vi "Periodic Tasks.vi"(8 "error in":errorcluster) -> ()   [LabVIEW 2018]
doc: "This VI runs in parallel to other tasks. It can contain as many user-defined periodic loops as you need. These can carry out PID or other sorts of timed response."
uses:
  <vilib>/Rock Robotics/WPI/ThirdParty/Sensors/navX/_TypeDefs/FRIC_navX_DeviceNumbersTypeDef.ctl
  <vilib>/Rock Robotics/WPI/DriverStation/WPI_DriverStationRobotMode2.ctl
  <vilib>/Rock Robotics/WPI/Solenoid/WPI_SolenoidValue.ctl
  <vilib>/Rock Robotics/WPI/Utilities/WPI_GetSetVariantRefNum.vi
  Robot Global Data.vi
  <vilib>/addons/control/pid/pid.llb/PID Control Input Filter (DBL).vi
  <vilib>/Rock Robotics/Network Tables/NT Write Boolean.vi
  <vilib>/Rock Robotics/WPI/RobotDrive/WPI_RobotDriveArcadeDrive_Standard(NoSaturation).vi
  <vilib>/Rock Robotics/WPI/Solenoid/WPI_SolenoidSetEnum.vi
  <vilib>/regexp/Match Regular Expression.xnode
  <vilib>/addons/control/pid/NI_PID_pid.lvlib
  <vilib>/addons/control/pid/pid.llb/PID (DBL).vi
panel:
  out "element 5":bool
  out "element 4":bool
  out "element 3":bool
  out "element 2":bool
  in  "Stage2_Speed":dbl=0.75
  in  "Stage1_Speed":dbl=0.75
  in  "ElevatorLowerBounds":dbl
  in  "ElevatorUpperBoundes":dbl
  in  "RotationEncoder_TopBall":dbl format="%#_13g"
  in  "Stage2Encoder_TopBall":dbl format="%#_13g"
  in  "Stage1Encoder_TopBall":dbl format="%#_13g"
  in  "RotationEncoder_TopHatch":dbl format="%#_13g"
  in  "Stage2Encoder_TopHatch":dbl format="%#_13g"
  in  "Stage1Encoder_TopHatch":dbl format="%#_13g"
  in  "RotationEncoder_MedBall":dbl format="%#_13g"
  in  "Stage2Encoder_MedBall":dbl format="%#_13g"
  in  "Stage1Encoder_MedBall":dbl format="%#_13g"
  in  "RotationEncoder_MedHatch":dbl format="%#_13g"
  in  "Stage2Encoder_MedHatch":dbl format="%#_13g"
  in  "Stage1Encoder_MedHatch":dbl format="%#_13g"
  in  "RotationEncoder_CargoBall":dbl format="%#_13g"
  in  "Stage2Encoder_CargoBall":dbl format="%#_13g"
  in  "Stage1Encoder_CargoBall":dbl format="%#_13g"
  in  "RotationEncoder_LowRocketBall":dbl format="%#_13g"
  in  "Stage2Encoder_LowRocketBall":dbl format="%#_13g"
  in  "Stage1Encoder_LowRocketBall":dbl format="%#_13g"
  in  "RotationEncoder_LowHatch":dbl format="%#_13g"
  in  "Stage2Encoder_LowHatch":dbl format="%#_13g"
  in  "Stage1Encoder_LowHatch":dbl format="%#_13g"
  in  "RotationEncoder_StartPosition":dbl format="%#_13g"
  in  "Stage2Encoder_StartPosition":dbl format="%#_13g"
  in  "Stage1Encoder_StartPosition":dbl format="%#_13g"
  out "stage 1 encoder":dbl
  in  "Stage1_EncoderReset":bool
  in  "driveMultiplier":dbl=1.0
  in  "rotationMultiplier":dbl=0.7
  out "stage 2 encoder":dbl
  in  "Stage2_EnconderReset":bool
  out "YRPHfH":T1
  in  "Update":bool
  in  "Device Number":T2
  in  "Pug Mode":bool
  out "error out":errorcluster
  in  "Reset Enconder Arm":bool
  out "Arm Encoder":dbl
  in  "Shooter Speed":dbl
  # "Motor Speed Controls:"
  # "Arm Rotation Control Variable:"
  # "LIFT AND ARM CONTROLS:"
  # "DRIVE SYSTEMS:"
  # "Lift and Arm Encoder Positions"
  # "This is the multiplier associated with the drive train's forward and backwards speed. You want this number to be possitive and between 0 and 1"
  # "This is the multiplier associated with the drive train's rotation. You want this number to be possitive and between 0 and 1"
  # "PID Control for drivetrain. It would essentially act as\na stay put for the robot. This would, in theory, fight\nback against another robot's defense with equal force\nhelping to stablize the robot."
  # "TESTING:"
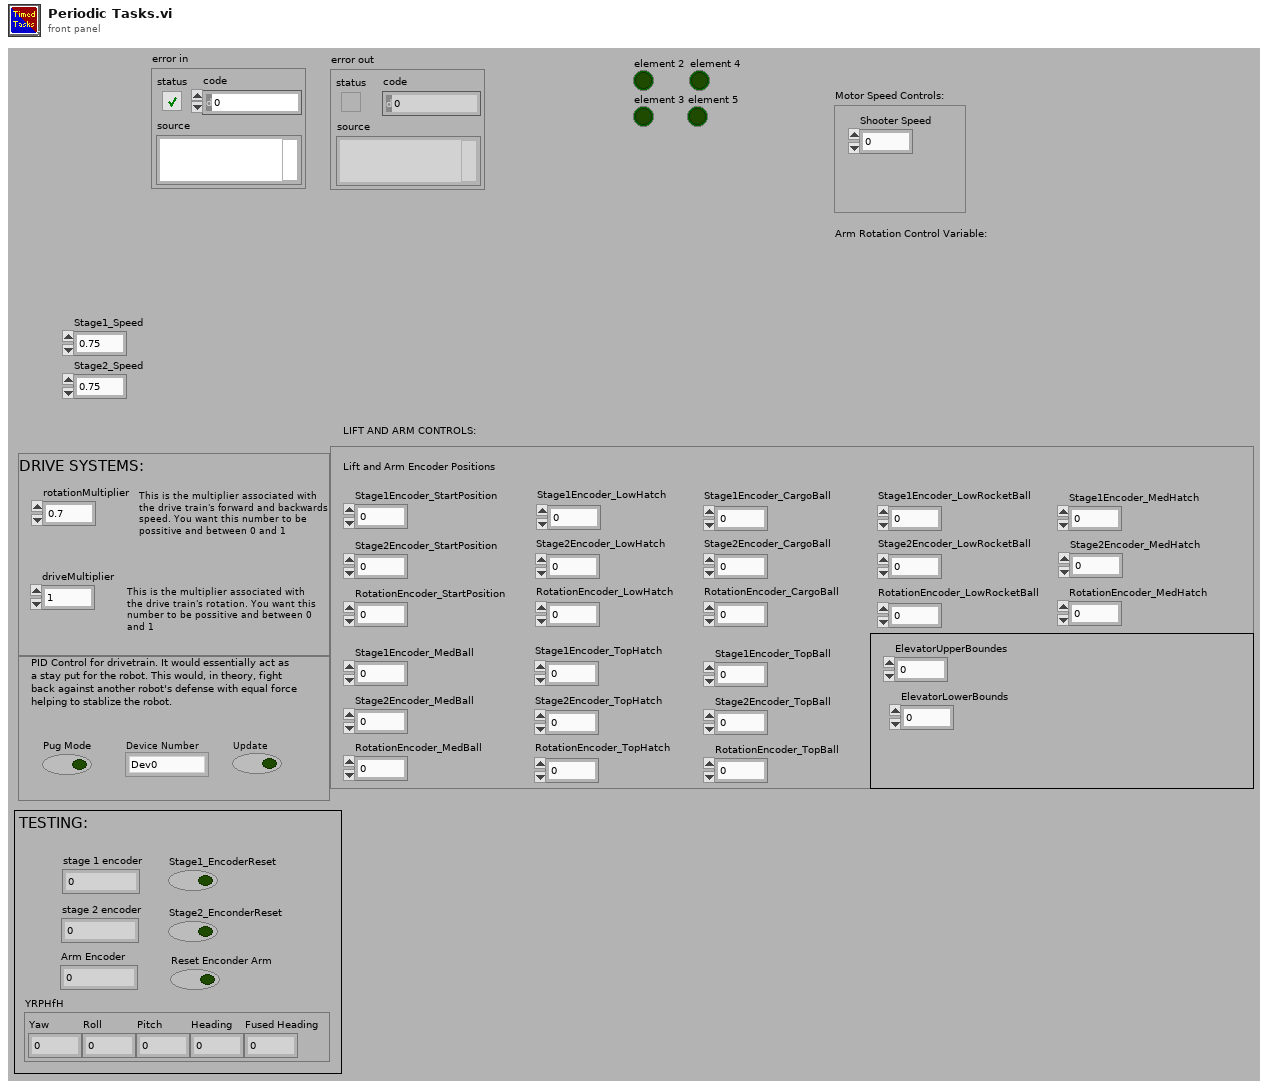
[diagram p1: front panel]
types:
  T1 = cluster{"Yaw":dbl, "Roll":dbl, "Pitch":dbl, "Heading":dbl, "Fused Heading":dbl}
  T2 = typedef "FRIC_navX_DeviceNumbersTypeDef.ctl" = enum16{"Dev0", "Dev1", "Dev2", "Dev3"}
  T3 = typedef "WPI_JoystickDevRef.ctl" = cluster{"Device":T4}
  T4 = typedef "WPI_JoystickDeviceEnum.ctl" = enum16{"USB 0", "USB 1", "USB 2", "USB 3", "USB 4", "USB 5"}
  T5 = typedef "WPI_RobotDriveDevRef.ctl" = cluster{"DevStatus":errorcluster, "Motors[]":T6[], "Square Inputs":bool, "Max Output":dbl}
  T6 = typedef "WPI_MotorControlDeviceRef.ctl" = cluster{"DeviceStatus":errorcluster, "Type":T7, "PWM":cluster{"PWM Channel":T8, "DeadBand":T9}, "CAN":cluster{"Device Number":u8, "SetOutput VI Ref":variant, "GetOutput VI Ref":variant, "Enable VI Ref":variant, "Disable VI Ref":variant, "Data":variant}, "Invert":bool, "DIO PWM":cluster{"PWM \"Enable\" Channel":T8, "DIOChannel":T10, "PWM Rate":dbl}}
  T7 = typedef "WPI_MotorControlType.ctl" = enum16{"PWM", "CAN", "DIO PWM"}
  T8 = typedef "FPGA_DIOPWMChannel.ctl" = enum8{"PWM 0", "PWM 1", "PWM 2", "PWM 3", "PWM 4", "PWM 5", "PWM 6", "PWM 7", "PWM 8", "PWM 9", "PWM MXP 0", "PWM MXP 1", "PWM MXP 2", "PWM MXP 3", "PWM MXP 4", "PWM MXP 5", "PWM MXP 6", "PWM MXP 7", "PWM MXP 8", "PWM MXP 9", "Invalid"}
  T9 = typedef "WPI_PWMDeadband.ctl" = cluster{"Name":string, "maxPositivePwm":i32, "minPositivePwm":i32, "centerPwm":i32, "maxNegativePwm":i32, "minNegativePwm":i32, "angularRange":u16}
  T10 = typedef "FPGA_DIOChannel.ctl" = enum8{"DIO 0", "DIO 1", "DIO 2", "DIO 3", "DIO 4", "DIO 5", "DIO 6", "DIO 7", "DIO 8", "DIO 9", "DIO MXP 0", "DIO MXP 1", "DIO MXP 2", "DIO MXP 3", "DIO MXP 4", "DIO MXP 5", "DIO MXP 6", "DIO MXP 7", "DIO MXP 8", "DIO MXP 9", "DIO MXP 10", "DIO MXP 11", "DIO MXP 12", "DIO MXP 13", "DIO MXP 14", "DIO MXP 15", "SPI Port CS1", "SPI Port CS2", "SPI Port CS3", "SPI Port MISO", "SPI Port MOSI", "Invalid"}
  T11 = typedef "WPI_EncoderDevRef.ctl" = cluster{"DevStatus":errorcluster, "EncoderIndex":T12, "CounterIndex":T13, "DistancePerCount":dbl, "Decoding Type":T14}
  T12 = typedef "FPGA_EncoderIdx.ctl" = enum8{"Enc 0", "Enc 1", "Enc 2", "Enc 3", "Enc 4", "Enc 5", "Enc 6", "Enc 7", "Invalid"}
  T13 = typedef "FPGA_CounterCtrSystemIndex.ctl" = enum8{"Ctr 0", "Ctr 1", "Ctr 2", "Ctr 3", "Ctr 4", "Ctr 5", "Ctr 6", "Ctr 7", "Invalid"}
  T14 = typedef "WPI_EncoderType.ctl" = enum16{"1x", "2x", "4x"}
  T15 = typedef "WPI_SolenoidDevRef.ctl" = cluster{"DevStatus":errorcluster, "Pneumatics Control Module":u8, "Forward Solenoid Channel":T16, "Reverse Solenoid Channel":T16}
  T16 = typedef "WPI_SolenoidChannel.ctl" = enum8{"Solenoid 0", "Solenoid 1", "Solenoid 2", "Solenoid 3", "Solenoid 4", "Solenoid 5", "Solenoid 6", "Solenoid 7", "Invalid"}
  T17 = typedef "WPI_DriverStationRobotMode2.ctl" = enum16{"Autonomous Disabled", "Autonomous Enabled", "Teleop Disabled", "Teleop Enabled", "Disconnected", "Finish", "Test Disabled", "Test Enabled", "Emergency Stopped"}
  T18 = typedef "WPI_SolenoidValue.ctl" = enum16{"Off", "On", "Forward", "Reverse"}
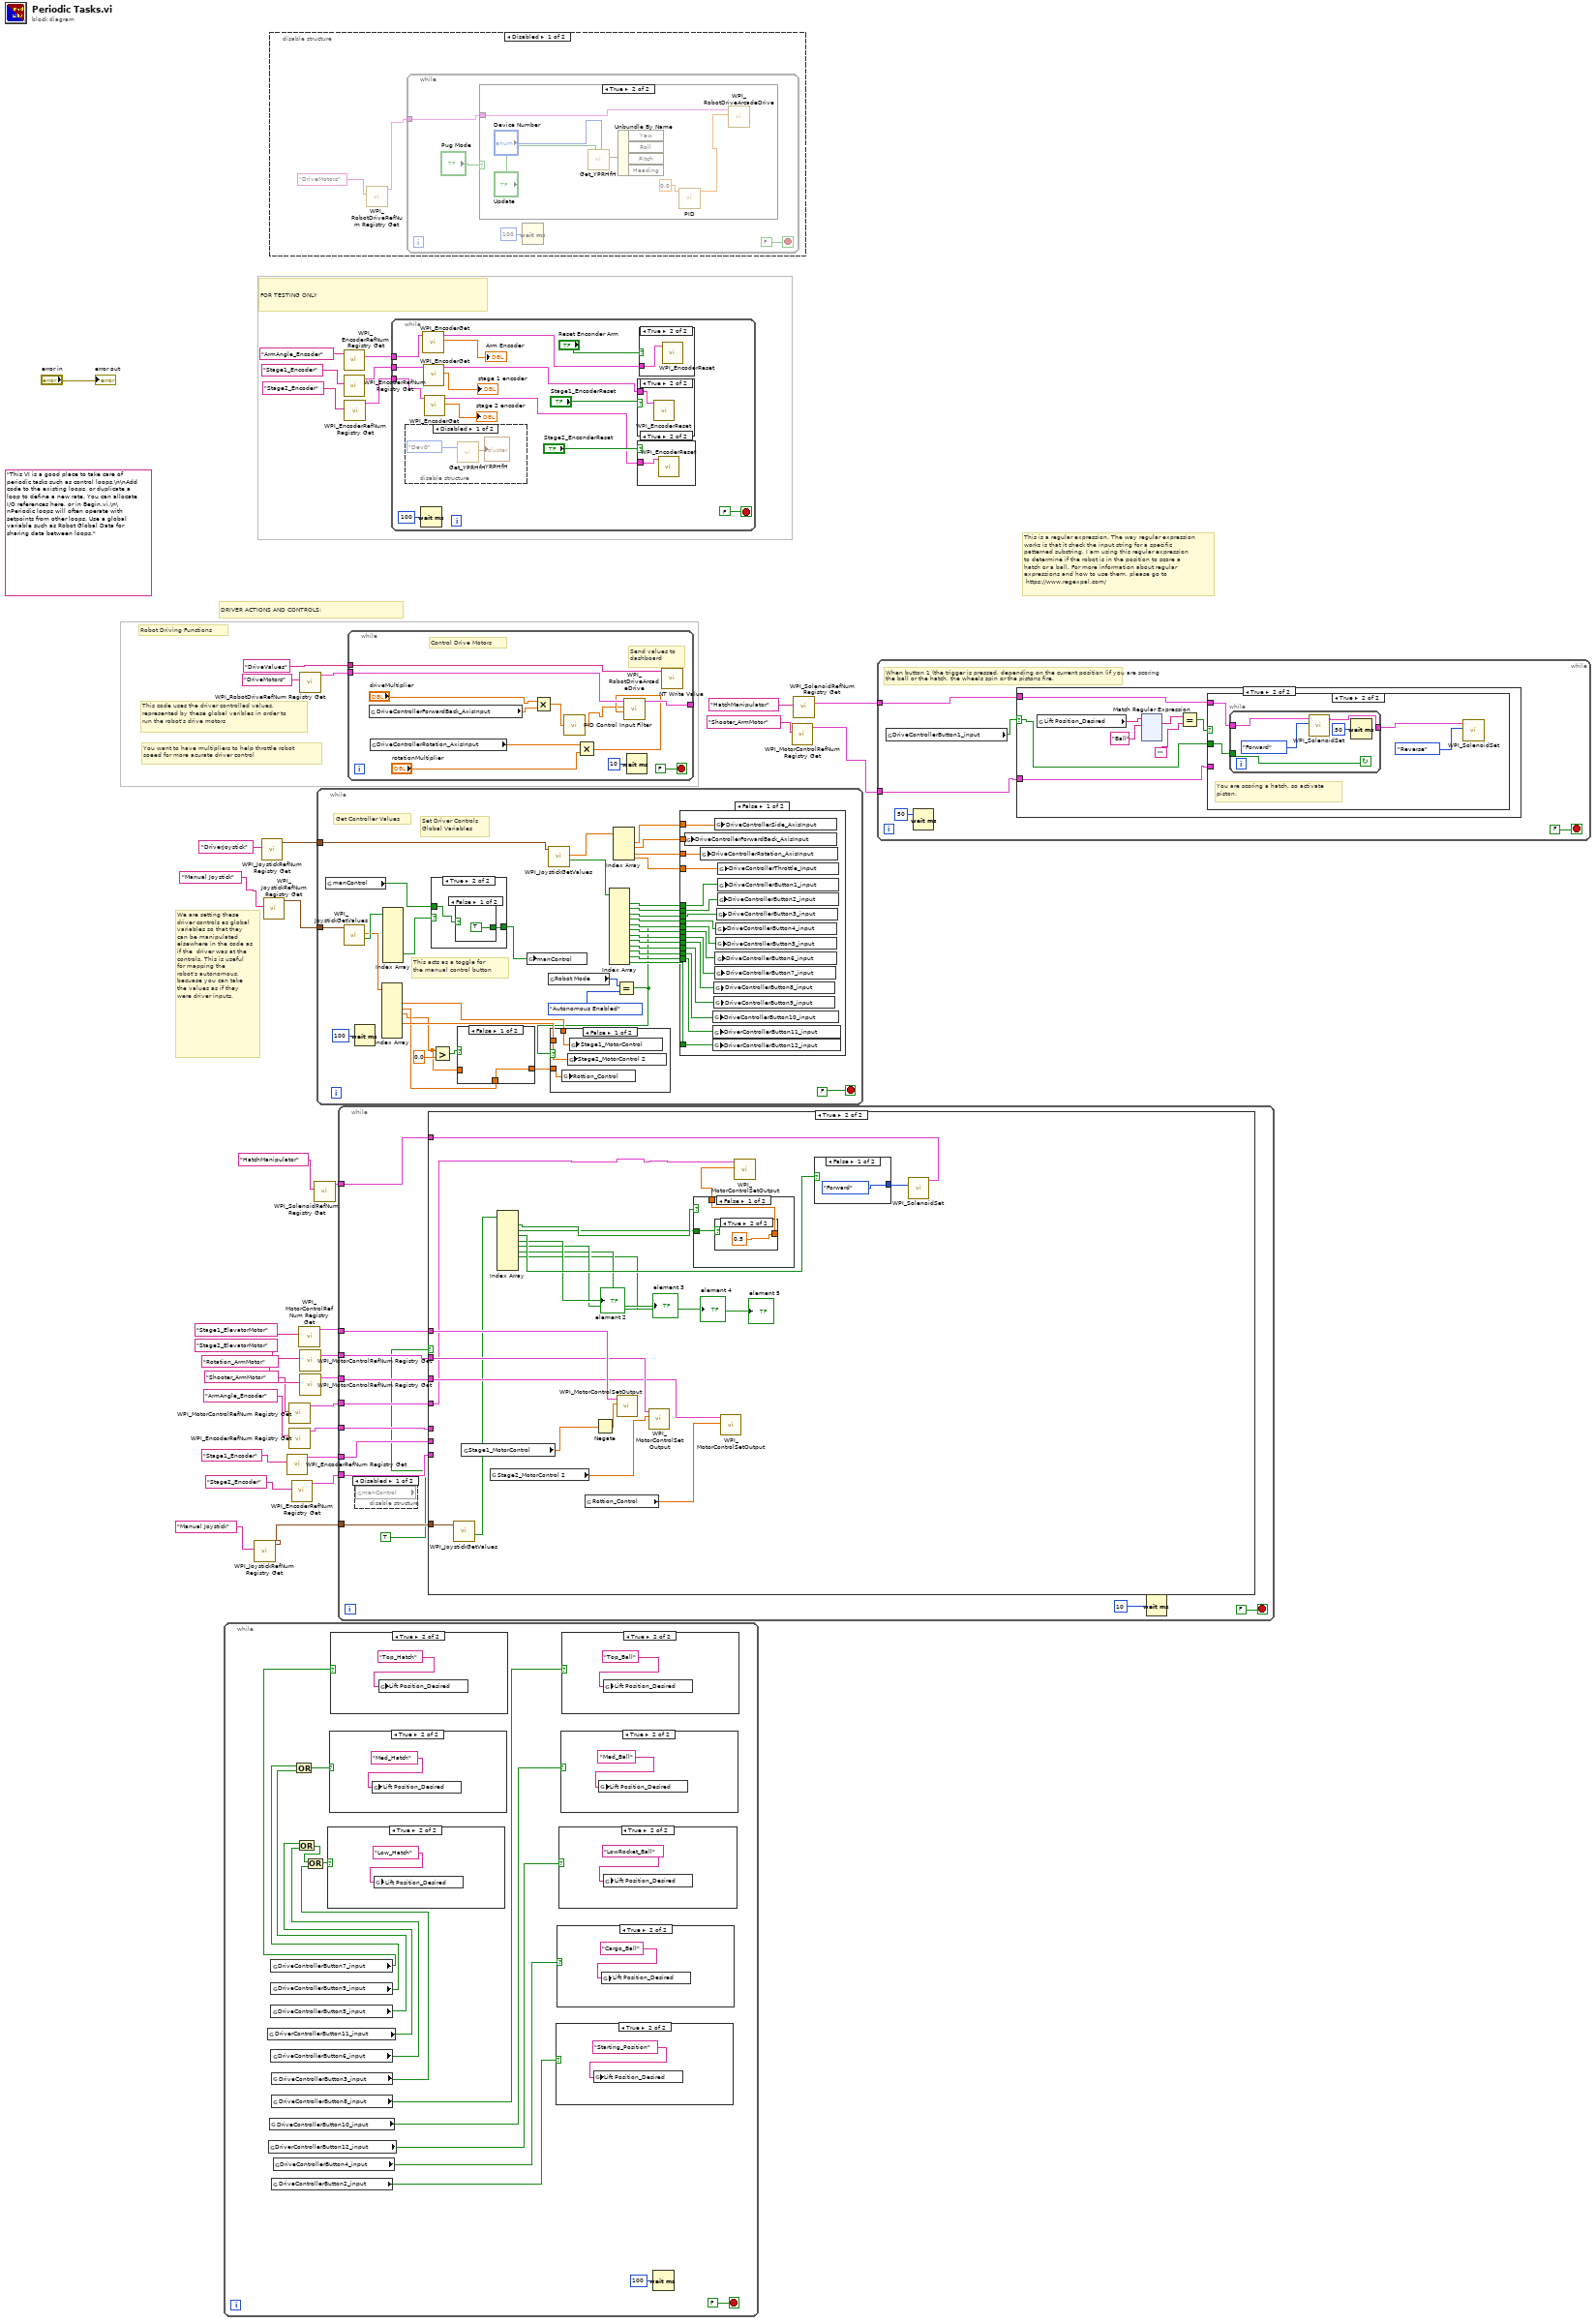
[diagram p0: block diagram]
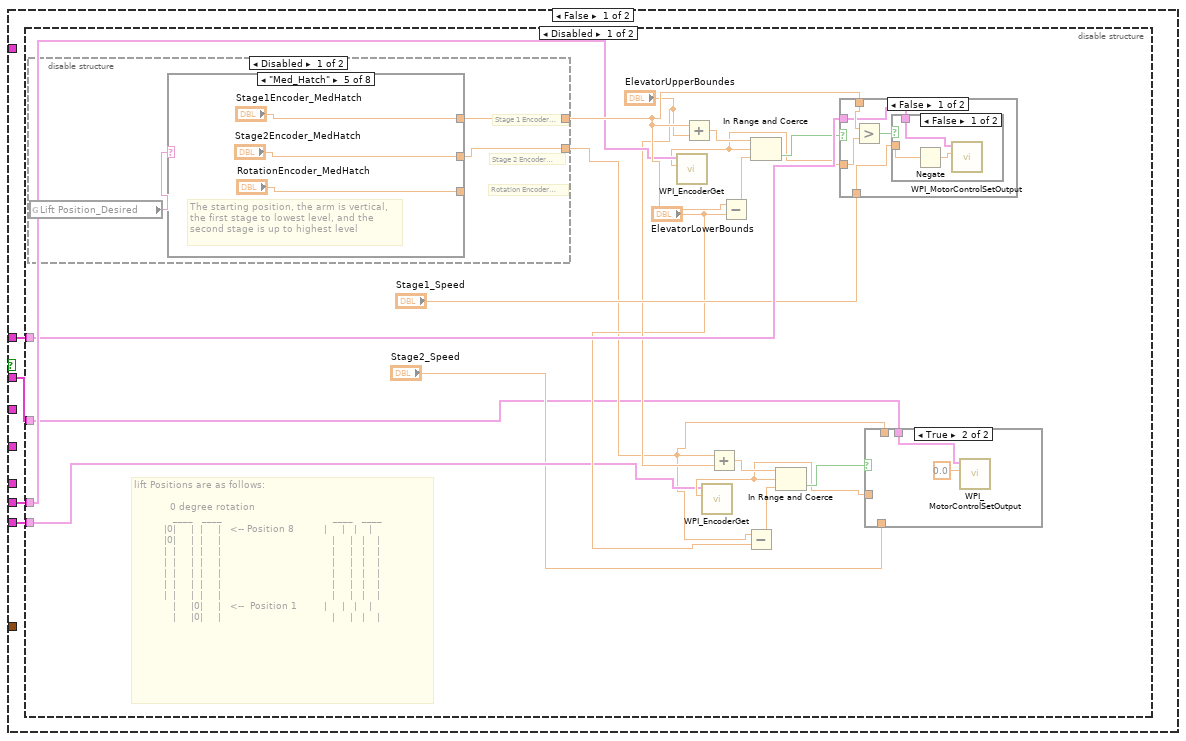
[diagram p3: hidden frame]
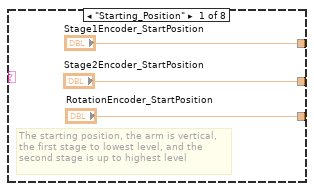
[diagram p4: hidden frame]
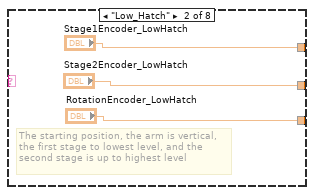
[diagram p5: hidden frame]
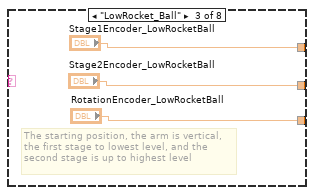
[diagram p6: hidden frame]
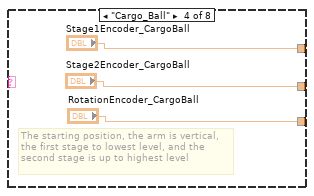
[diagram p7: hidden frame]
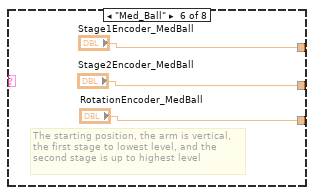
[diagram p8: hidden frame]
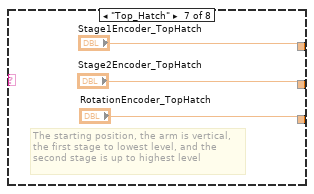
[diagram p9: hidden frame]
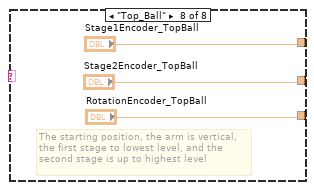
[diagram p10: hidden frame]
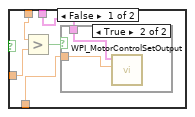
[diagram p12: hidden frame]
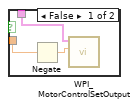
[diagram p13: hidden frame]
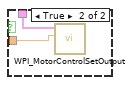
[diagram p14: hidden frame]
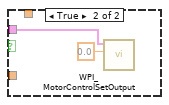
[diagram p15: hidden frame]
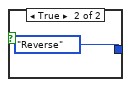
[diagram p17: hidden frame]
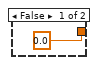
[diagram p18: hidden frame]
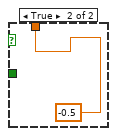
[diagram p19: hidden frame]
diagram:
  (unwired) "This VI is a good place to take care of periodic tasks such as control loops.\n\nAdd code to the existing loops, or duplicate a loop to define a new rate. You can allocate I/O references here, or in Begin.vi.\n\nPeriodic loops will often operate with setpoints from other loops. Use a global variable such as Robot Global Data for sharing data between loops."
  # "We are setting these driver controls as global variables so that they can be manipulated elsewhere in the code as if the  driver was at the controls. This is useful for mapping the\nrobot's autonomous, becuase you can take\nthe values as if they were driver inputs."
  # "You want to have multipliers to help throttle robot\nsoeed for more acurate driver control"
  # "This code uses the driver controlled values,\nrepresented by these global varibles in order to\nrun the robot's drive motors"
  # "FOR TESTING ONLY"
  # "This is a regular expression. The way regular expression\nworks is that it check the input string for a specific\npatterned substring. I am using this regular expression\nto determine if the robot is in the position to score a \nhatch or a ball. For more information about regular\nexpressions and how to use them, please go to\n https://www.regexpal.com/"
  # "Robot Driving Functions"
  # "DRIVER ACTIONS AND CONTROLS:"
  n1 = while {
    stop <- FALSE stop-if-true
    n2 = global read "Robot Global Data.vi" "DriverControllerButton11_input"() -> (w47:bool)
    n3 = global read "Robot Global Data.vi" "DriverControllerButton12_input"() -> (w41:bool)
    n4 = global read "Robot Global Data.vi" "DriveControllerButton10_input"() -> (w42:bool)
    n5 = global read "Robot Global Data.vi" "DriveControllerButton7_input"() -> (w51:bool)
    n6 = global read "Robot Global Data.vi" "DriveControllerButton9_input"() -> (w49:bool)
    n7 = global read "Robot Global Data.vi" "DriveControllerButton5_input"() -> (w48:bool)
    n8 = global read "Robot Global Data.vi" "DriveControllerButton6_input"() -> (w46:bool)
    n9 = global read "Robot Global Data.vi" "DriveControllerButton3_input"() -> (w37:bool)
    n10 = global read "Robot Global Data.vi" "DriveControllerButton8_input"() -> (w43:bool)
    n11 = global read "Robot Global Data.vi" "DriveControllerButton2_input"() -> (w44:bool)
    n12 = global read "Robot Global Data.vi" "DriveControllerButton4_input"() -> (w40:bool)
    n13 = Or(x=w49, y=w48) -> (x .or. y?=w50:bool)
    n14 = Or(x=w47, y=w46) -> (x .or. y?=w38:bool)
    n15 = Or(x=w38, y=w37) -> (x .or. y?=w45:bool)
    n16 = case shown="True" w45 {
      frame False {
      }
      frame True {
        n17 = global write "Robot Global Data.vi" "Lift Position_Desired"("Low_Hatch") -> ()
      }
    }
    n18 = case shown="True" w50 {
      frame False {
      }
      frame True {
        n19 = global write "Robot Global Data.vi" "Lift Position_Desired"("Med_Hatch") -> ()
      }
    }
    n20 = case shown="True" w51 {
      frame False {
      }
      frame True {
        n21 = global write "Robot Global Data.vi" "Lift Position_Desired"("Top_Hatch") -> ()
      }
    }
    n22 = case shown="True" w44 {
      frame False {
      }
      frame True {
        n23 = global write "Robot Global Data.vi" "Lift Position_Desired"("Starting_Position") -> ()
      }
    }
    n24 = case shown="True" w40 {
      frame False {
      }
      frame True {
        n25 = global write "Robot Global Data.vi" "Lift Position_Desired"("Cargo_Ball") -> ()
      }
    }
    n26 = case shown="True" w41 {
      frame False {
      }
      frame True {
        n27 = global write "Robot Global Data.vi" "Lift Position_Desired"("LowRocket_Ball") -> ()
      }
    }
    n28 = case shown="True" w42 {
      frame False {
      }
      frame True {
        n29 = global write "Robot Global Data.vi" "Lift Position_Desired"("Med_Ball") -> ()
      }
    }
    n30 = case shown="True" w43 {
      frame False {
      }
      frame True {
        n31 = global write "Robot Global Data.vi" "Lift Position_Desired"("Top_Ball") -> ()
      }
    }
    n32 = Wait (ms)(milliseconds to wait=u32 100) -> ()  [unwired: 1 out]
  }
  n33 = call <vilib>:"WPI_JoystickRefNum Registry Get.vi"("refnum name"="Manual Joystick") -> ("JoystickDevRef"=w24:T3)  [unwired: 9 in, 1 out]
  n34 = call <vilib>:"WPI_JoystickRefNum Registry Get.vi"("refnum name"="DriverJoystick") -> ("JoystickDevRef"=w32:T3)  [unwired: 9 in, 1 out]
  n35 = call <vilib>:"WPI_JoystickRefNum Registry Get.vi"("refnum name"="Manual Joystick") -> ("JoystickDevRef"=w21:T3)  [unwired: 9 in, 1 out]
  n36 = disable-structure shown="Disabled" {
    frame Disabled {
      n37 = call <vilib>:"WPI_RobotDriveRefNum Registry Get.vi"("refnum name"="DriveMotors") -> ("RobotDriveDevRef"=w61:T5)  [unwired: 9 in, 1 out]
      n38 = while {
        tunnel: w61 -> [w63]
        stop <- FALSE stop-if-true
        n39 = case shown="True" "Pug Mode" {
          tunnel: w63 -> [_ w69]
          frame False {
          }
          frame True {
            n40 = call <vilib>:"Get_YPRHfH.vi"("Device Number"="Device Number", "Update"="Update") -> ("YRPHfH"=w72:T1)  [unwired: 9 in]
            n41 = Unbundle By Name(w72) -> ()  [unwired: 4 out]
            n42 = call-poly <vilib>:"PID.vi"("setpoint"=0.0) -> ("output"=w68:dbl)  [unwired: 9 in, 1 out]
            n43 = call-poly <vilib>:"WPI_RobotDriveArcadeDrive.vi"("X axis value"=w68, "RobotDriveDevRef"=w69) -> ()  [unwired: 7 in, 3 out]
          }
        }
        n44 = Wait (ms)(milliseconds to wait=u32 100) -> ()  [unwired: 1 out]
      }
    }
    frame Enabled {
    }
  }
  n45 = call <vilib>:"WPI_EncoderRefNum Registry Get.vi"("refnum name"="Stage1_Encoder") -> ("EncoderDevRef"=w4:T11)  [unwired: 9 in, 1 out]
  n46 = call <vilib>:"WPI_MotorControlRefNum Registry Get.vi"("refnum name"="Shooter_ArmMotor") -> ("MotorControlDevRef"=w11:T6)  [unwired: 9 in, 1 out]
  n47 = call <vilib>:"WPI_EncoderRefNum Registry Get.vi"("refnum name"="ArmAngle_Encoder") -> ("EncoderDevRef"=w10:T11)  [unwired: 9 in, 1 out]
  n48 = call <vilib>:"WPI_EncoderRefNum Registry Get.vi"("refnum name"="Stage2_Encoder") -> ("EncoderDevRef"=w9:T11)  [unwired: 9 in, 1 out]
  n49 = call <vilib>:"WPI_MotorControlRefNum Registry Get.vi"("refnum name"="Stage1_ElevatorMotor") -> ("MotorControlDevRef"=w14:T6)  [unwired: 9 in, 1 out]
  n50 = call <vilib>:"WPI_RobotDriveRefNum Registry Get.vi"("refnum name"="DriveMotors") -> ("RobotDriveDevRef"=w36:T5)  [unwired: 9 in, 1 out]
  n51 = call <vilib>:"WPI_MotorControlRefNum Registry Get.vi"("refnum name"="Stage2_ElevatorMotor") -> ("MotorControlDevRef"=w13:T6)  [unwired: 9 in, 1 out]
  n52 = call <vilib>:"WPI_MotorControlRefNum Registry Get.vi"("refnum name"="Rotation_ArmMotor") -> ("MotorControlDevRef"=w12:T6)  [unwired: 9 in, 1 out]
  n53 = call <vilib>:"WPI_SolenoidRefNum Registry Get.vi"("refnum name"="HatchManipulator") -> ("SolenoidDevRef"=w22:T15)  [unwired: 9 in, 1 out]
  n54 = while {
    tunnel: w32 -> [w109]
    tunnel: w21 -> [w102]
    stop <- FALSE stop-if-true
    # "This acts as a toggle for \nthe manual control button"
    # "Set Driver Controls\nGlobal Variables"
    # "Get Controller Values"
    n55 = global read "Robot Global Data.vi" "manControl"() -> (w100:bool)
    n56 = call <vilib>:"WPI_JoystickGetValues.vi"("JoystickDevRef"=w102) -> ("Buttons"=w101:bool[], "Axes"=w81:dbl[])  [unwired: 6 in, 3 out]
    n57 = Wait (ms)(milliseconds to wait=u32 100) -> ()  [unwired: 1 out]
    n58 = Index Array(array=w81) -> (element #2=w74:dbl, element #3=w77:dbl, element #4=w76:dbl, element #6=w80:dbl)  [unwired: 8 in, 4 out]
    n59 = Index Array(array=w101) -> (element #7=w84:bool)  [unwired: 8 in, 7 out]
    n60 = case shown="True" w84 {
      tunnel: w100 -> [w132 w133]
      tunnel: [w132 w134] -> w99
      frame False {
      }
      frame True {
        n61 = case shown="False" w133 {
          tunnel: [TRUE FALSE] -> w134
          frame False {
          }
          frame True {
          }
        }
      }
    }
    n62 = Greater?(x=w76, y=0.0) -> (0:w79:bool)
    n63 = case shown="False" w79 {
      tunnel: w76 -> [_ w115]
      tunnel: [w113 w114] -> w75
      tunnel: w77 -> [w113 _]
      frame False {
      }
      frame True {
        n64 = Negate(x=w115) -> (-x=w114:dbl)
      }
    }
    n65 = global write "Robot Global Data.vi" "manControl"(w99) -> ()
    n66 = global read "Robot Global Data.vi" "Robot Mode"() -> (w83:T17)
    n67 = call <vilib>:"WPI_JoystickGetValues.vi"("JoystickDevRef"=w109) -> ("Buttons"=w107:bool[], "Axes"=w108:dbl[])  [unwired: 6 in, 3 out]
    n68 = Index Array(array=w107) -> (element #1=w86:bool, element #2=w87:bool, element #3=w88:bool, element #4=w89:bool, element #5=w90:bool, element #6=w91:bool, element #7=w92:bool, element #8=w94:bool, element #9=w93:bool, element #10=w95:bool, element #11=w96:bool, element #12=w97:bool)  [unwired: 12 in]
    n69 = Index Array(array=w108) -> (element #1=w85:dbl, element #2=w103:dbl, element #3=w106:dbl, element #4=w105:dbl)  [unwired: 4 in]
    n70 = Equal?(x=w83, y=WPI_DriverStationRobotMode2."Autonomous Enabled") -> (x = y?=w73:bool)
    n71 = case shown="False" w73 {
      tunnel: w80 -> [w112 _]
      tunnel: w75 -> [w111 _]
      tunnel: w74 -> [w110 _]
      frame False {
        n72 = global write "Robot Global Data.vi" "Rottion_Control"(w111) -> ()
        n73 = global write "Robot Global Data.vi" "Stage2_MotorControl 2"(w112) -> ()
        n74 = global write "Robot Global Data.vi" "Stage1_MotorControl"(w110) -> ()
      }
      frame True {
      }
    }
    n75 = case shown="False" w73 {
      tunnel: w106 -> [w131 _]
      tunnel: w105 -> [w130 _]
      tunnel: w103 -> [w129 _]
      tunnel: w97 -> [w128 _]
      tunnel: w96 -> [w127 _]
      tunnel: w95 -> [w126 _]
      tunnel: w94 -> [w125 _]
      tunnel: w93 -> [w124 _]
      tunnel: w92 -> [w123 _]
      tunnel: w91 -> [w122 _]
      tunnel: w90 -> [w121 _]
      tunnel: w89 -> [w120 _]
      tunnel: w88 -> [w119 _]
      tunnel: w87 -> [w118 _]
      tunnel: w86 -> [w117 _]
      tunnel: w85 -> [w116 _]
      frame False {
        n76 = global write "Robot Global Data.vi" "DriveControllerForwardBack_AxisInput"(w129) -> ()
        n77 = global write "Robot Global Data.vi" "DriveControllerRotation_AxisInput"(w131) -> ()
        n78 = global write "Robot Global Data.vi" "DriveControllerButton10_input"(w126) -> ()
        n79 = global write "Robot Global Data.vi" "DriverControllerButton11_input"(w127) -> ()
        n80 = global write "Robot Global Data.vi" "DriverControllerButton12_input"(w128) -> ()
        n81 = global write "Robot Global Data.vi" "DriveControllerButton8_input"(w125) -> ()
        n82 = global write "Robot Global Data.vi" "DriveControllerButton9_input"(w124) -> ()
        n83 = global write "Robot Global Data.vi" "DriveControllerSide_AxisInput"(w116) -> ()
        n84 = global write "Robot Global Data.vi" "DriveControllerButton7_input"(w123) -> ()
        n85 = global write "Robot Global Data.vi" "DriveControllerButton6_input"(w122) -> ()
        n86 = global write "Robot Global Data.vi" "DriveControllerButton4_input"(w120) -> ()
        n87 = global write "Robot Global Data.vi" "DriveControllerButton5_input"(w121) -> ()
        n88 = global write "Robot Global Data.vi" "DriveControllerButton3_input"(w119) -> ()
        n89 = global write "Robot Global Data.vi" "DriveControllerButton2_input"(w118) -> ()
        n90 = global write "Robot Global Data.vi" "DriveControllerThrottle_Input"(w130) -> ()
        n91 = global write "Robot Global Data.vi" "DriveControllerButton1_input"(w117) -> ()
      }
      frame True {
      }
    }
  }
  n92 = while {
    tunnel: w14 -> [w148]
    tunnel: w13 -> [w139]
    tunnel: w12 -> [w147]
    tunnel: w24 -> [w146]
    tunnel: w22 -> [w145]
    tunnel: w9 -> [w144]
    tunnel: w10 -> [w143]
    tunnel: w11 -> [w142]
    tunnel: w4 -> [w138]
    stop <- FALSE stop-if-true
    n93 = disable-structure shown="Disabled" {
      frame Disabled {
        n94 = global read "Robot Global Data.vi" "manControl"() -> ()  [unwired: 1 out]
      }
      frame Enabled {
      }
    }
    n95 = case shown="True" TRUE {
      tunnel: w148 -> [w151 w240]
      tunnel: w139 -> [w149 w239]
      tunnel: w147 -> [_ w238]
      tunnel: w142 -> [_ w226]
      tunnel: w143 -> [_ _]
      tunnel: w144 -> [w150 _]
      tunnel: w146 -> [_ w241]
      tunnel: w145 -> [_ w236]
      tunnel: w138 -> [w152 _]
      frame False {
        n96 = disable-structure shown="Disabled" {
          disable-tunnel: w152 -> [w169 _]
          disable-tunnel: w151 -> [w168 _]
          disable-tunnel: w150 -> [w156 _]
          disable-tunnel: w149 -> [w153 _]
          frame Disabled {
            # "lift Positions are as follows:\n\n            0 degree rotation\n             ____   ____                                     ____   ____     \n          |0|     |  |     |   <-- Position 8          |     |   |    |                 \n          |0|     |  |     |                                     |     |   |    |\n          |  |     |  |     |                                     |     |   |    |\n          |  |     |  |     |                                     |     |   |    |\n          |  |     |  |     |                                     |     |   |    |\n          |  |     |  |     |                                     |     |   |    |\n          |  |     |  |     |                                     |     |   |    |\n             |     |0|     |   <--  Position 1         |     |   |    |\n             |     |0|     |                                     |     |   |    |"
            n97 = disable-structure shown="Disabled" {
              disable-tunnel: [w173 _] -> w170
              disable-tunnel: [w172 _] -> w155
              frame Disabled {
                # "Rotation Encoder Limit"
                # "Stage 2 Encoder Limit"
                # "Stage 1 Encoder Limit"
                n98 = global read "Robot Global Data.vi" "Lift Position_Desired"() -> (w171:string)
                n99 = case shown="\"Med_Hatch\"" w171 {
                  tunnel: ["Stage1Encoder_StartPosition" "Stage1Encoder_LowHatch" "Stage1Encoder_LowRocketBall" "Stage1Encoder_CargoBall" "Stage1Encoder_MedHatch" "Stage1Encoder_MedBall" "Stage1Encoder_TopHatch" "Stage1Encoder_TopBall"] -> w173
                  tunnel: ["Stage2Encoder_StartPosition" "Stage2Encoder_LowHatch" "Stage2Encoder_LowRocketBall" "Stage2Encoder_CargoBall" "Stage2Encoder_MedHatch" "Stage2Encoder_MedBall" "Stage2Encoder_TopHatch" "Stage2Encoder_TopBall"] -> w172
                  tunnel: ["RotationEncoder_StartPosition" "RotationEncoder_LowHatch" "RotationEncoder_LowRocketBall" "RotationEncoder_CargoBall" "RotationEncoder_MedHatch" "RotationEncoder_MedBall" "RotationEncoder_TopHatch" "RotationEncoder_TopBall"] -> _
                  frame "Starting_Position" {
                    # "The starting position, the arm is vertical,\nthe first stage to lowest level, and the\nsecond stage is up to highest level"
                  }
                  frame "Low_Hatch" {
                    # "The starting position, the arm is vertical,\nthe first stage to lowest level, and the\nsecond stage is up to highest level"
                  }
                  frame "LowRocket_Ball" {
                    # "The starting position, the arm is vertical,\nthe first stage to lowest level, and the\nsecond stage is up to highest level"
                  }
                  frame "Cargo_Ball" {
                    # "The starting position, the arm is vertical,\nthe first stage to lowest level, and the\nsecond stage is up to highest level"
                  }
                  frame "Med_Hatch" {
                    # "The starting position, the arm is vertical,\nthe first stage to lowest level, and the\nsecond stage is up to highest level"
                  }
                  frame "Med_Ball" {
                    # "The starting position, the arm is vertical,\nthe first stage to lowest level, and the\nsecond stage is up to highest level"
                  }
                  frame "Top_Hatch" {
                    # "The starting position, the arm is vertical,\nthe first stage to lowest level, and the\nsecond stage is up to highest level"
                  }
                  frame "Top_Ball" {
                    # "The starting position, the arm is vertical,\nthe first stage to lowest level, and the\nsecond stage is up to highest level"
                  }
                }
              }
              frame Enabled {
              }
            }
            n100 = call <vilib>:"WPI_EncoderGet.vi"("EncoderDevRef"=w169) -> ("Distance"=w163:dbl)  [unwired: 5 in, 5 out]
            n101 = Add(x=w170, y="ElevatorUpperBoundes") -> (x+y=w165:dbl)
            n102 = call <vilib>:"WPI_EncoderGet.vi"("EncoderDevRef"=w156) -> ("Distance"=w159:dbl)  [unwired: 5 in, 5 out]
            n103 = Add(x=w155, y="ElevatorUpperBoundes") -> (x+y=w161:dbl)
            n104 = Subtract(x=w170, y="ElevatorLowerBounds") -> (x-y=w164:dbl)
            n105 = Subtract(x=w155, y="ElevatorLowerBounds") -> (x-y=w160:dbl)
            n106 = In Range and Coerce(upper limit=w165, x=w163, lower limit=w164) -> (In Range?=w166:bool)  [unwired: 1 out]
            n107 = In Range and Coerce(upper limit=w161, x=w159, lower limit=w160) -> (In Range?=w162:bool)  [unwired: 1 out]
            n108 = case shown="False" w166 {
              tunnel: w168 -> [w211 w221]
              tunnel: "Stage1_Speed" -> [w210 _]
              tunnel: w170 -> [w213 _]
              tunnel: w163 -> [w212 _]
              frame False {
                n109 = Greater?(x=w213, y=w212) -> (0:w214:bool)
                n110 = case shown="False" w214 {
                  tunnel: w211 -> [w215 w219]
                  tunnel: w210 -> [w217 w218]
                  frame False {
                    n111 = Negate(x=w217) -> (-x=w216:dbl)
                    n112 = call <vilib>:"WPI_MotorControlSetOutput.vi"("Output"=w216, "MotorControlDevRef"=w215) -> ()  [unwired: 7 in, 3 out]
                  }
                  frame True {
                    n113 = call <vilib>:"WPI_MotorControlSetOutput.vi"("Output"=w218, "MotorControlDevRef"=w219) -> ()  [unwired: 7 in, 3 out]
                  }
                }
              }
              frame True {
                n114 = call <vilib>:"WPI_MotorControlSetOutput.vi"("Output"=0.0, "MotorControlDevRef"=w221) -> ()  [unwired: 7 in, 3 out]
              }
            }
            n115 = case shown="True" w162 {
              tunnel: "Stage2_Speed" -> [w199 _]
              tunnel: w155 -> [w201 _]
              tunnel: w159 -> [w200 _]
              tunnel: w153 -> [w198 w208]
              frame False {
                n116 = Greater?(x=w201, y=w200) -> (0:w202:bool)
                n117 = case shown="True" w202 {
                  tunnel: w199 -> [w205 w207]
                  tunnel: w198 -> [w203 w206]
                  frame False {
                    n118 = Negate(x=w205) -> (-x=w204:dbl)
                    n119 = call <vilib>:"WPI_MotorControlSetOutput.vi"("Output"=w204, "MotorControlDevRef"=w203) -> ()  [unwired: 7 in, 3 out]
                  }
                  frame True {
                    n120 = call <vilib>:"WPI_MotorControlSetOutput.vi"("Output"=w207, "MotorControlDevRef"=w206) -> ()  [unwired: 7 in, 3 out]
                  }
                }
              }
              frame True {
                n121 = call <vilib>:"WPI_MotorControlSetOutput.vi"("Output"=0.0, "MotorControlDevRef"=w208) -> ()  [unwired: 7 in, 3 out]
              }
            }
          }
          frame Enabled {
          }
        }
      }
      frame True {
        n122 = call <vilib>:"WPI_JoystickGetValues.vi"("JoystickDevRef"=w241) -> ("Buttons"=w237:bool[])  [unwired: 6 in, 4 out]
        n123 = global read "Robot Global Data.vi" "Stage1_MotorControl"() -> (w224:dbl)
        n124 = global read "Robot Global Data.vi" "Stage2_MotorControl 2"() -> (w223:dbl)
        n125 = Index Array(array=w237) -> (element #1=w227:bool, element #2=w225:bool, element #3=w233:bool, element #4=→"element 2":bool, element #5=→"element 3":bool, element #6=→"element 4":bool, element #7=→"element 5":bool)  [unwired: 9 in, 2 out]
        n126 = global read "Robot Global Data.vi" "Rottion_Control"() -> (w222:dbl)
        n127 = Negate(x=w224) -> (-x=w232:dbl)
        n128 = call <vilib>:"WPI_MotorControlSetOutput.vi"("Output"=w232, "MotorControlDevRef"=w240) -> ()  [unwired: 7 in, 3 out]
        n129 = call <vilib>:"WPI_MotorControlSetOutput.vi"("Output"=w223, "MotorControlDevRef"=w239) -> ()  [unwired: 7 in, 3 out]
        n130 = case shown="False" w227 {
          tunnel: [w245 -0.5 ("Output")] -> w235
          tunnel: w225 -> [w244 _]
          frame False {
            n131 = case shown="True" w244 {
              tunnel: [0.0 ("Output") 0.5 ("Output")] -> w245
              frame False {
              }
              frame True {
              }
            }
          }
          frame True {
          }
        }
        n132 = call <vilib>:"WPI_MotorControlSetOutput.vi"("Output"=w222, "MotorControlDevRef"=w238) -> ()  [unwired: 7 in, 3 out]
        n133 = call <vilib>:"WPI_MotorControlSetOutput.vi"("Output"=w235, "MotorControlDevRef"=w226) -> ()  [unwired: 7 in, 3 out]
        n134 = case shown="False" w233 {
          tunnel: [WPI_SolenoidValue."Forward" ("Value") WPI_SolenoidValue."Reverse" ("Value")] -> w234
          frame False {
          }
          frame True {
          }
        }
        n135 = call-poly <vilib>:"WPI_SolenoidSet.vi"("Value"=w234, "SolenoidDevRef"=w236) -> ()  [unwired: 8 in, 2 out]
      }
    }
    n136 = Wait (ms)(milliseconds to wait=u32 10) -> ()  [unwired: 1 out]
  }
  n137 = call <vilib>:"WPI_EncoderRefNum Registry Get.vi"("refnum name"="ArmAngle_Encoder") -> ("EncoderDevRef"=w27:T11)  [unwired: 9 in, 1 out]
  n138 = call <vilib>:"WPI_EncoderRefNum Registry Get.vi"("refnum name"="Stage1_Encoder") -> ("EncoderDevRef"=w6:T11)  [unwired: 9 in, 1 out]
  n139 = call <vilib>:"WPI_EncoderRefNum Registry Get.vi"("refnum name"="Stage2_Encoder") -> ("EncoderDevRef"=w7:T11)  [unwired: 9 in, 1 out]
  n140 = while {
    tunnel: w36 -> [w259]
    tunnel: [w258] -> _
    tunnel: "DriveValues" ("Name") -> [w257]
    stop <- FALSE stop-if-true
    # "Send values to \ndashboard"
    # "Control Drive Motors"
    n141 = global read "Robot Global Data.vi" "DriveControllerForwardBack_AxisInput"() -> (w251:dbl)
    n142 = global read "Robot Global Data.vi" "DriveControllerRotation_AxisInput"() -> (w255:dbl)
    n143 = Multiply(x="driveMultiplier", y=w251) -> (x*y=w250:dbl)
    n144 = call-poly <vilib>:"PID Control Input Filter.vi"("input"=w250) -> ("output"=w249:dbl)  [unwired: 4 in]
    n145 = Multiply(x=w255, y="rotationMultiplier") -> (x*y=w253:dbl)
    n146 = call-poly <vilib>:"WPI_RobotDriveArcadeDrive.vi"("Y axis value"=w253, "X axis value"=w249, "RobotDriveDevRef"=w259) -> ("RobotDriveDevRef"=w258:T5)  [unwired: 6 in, 2 out]
    n147 = Wait (ms)(milliseconds to wait=u32 10) -> ()  [unwired: 1 out]
    n148 = call-poly <vilib>:"NT Write Value.vi"("Name"=w257) -> ()  [unwired: 10 in, 1 out]
  }
  n149 = while {
    tunnel: w27 -> [w272]
    tunnel: w7 -> [w263]
    tunnel: w6 -> [w268]
    stop <- FALSE stop-if-true
    n150 = disable-structure shown="Disabled" {
      frame Disabled {
        n151 = call <vilib>:"Get_YPRHfH.vi"("Device Number"=FRIC_navX_DeviceNumbersTypeDef."Dev0") -> ("YRPHfH"=→"YRPHfH":T1)  [unwired: 10 in]
      }
      frame Enabled {
      }
    }
    n152 = Wait (ms)(milliseconds to wait=u32 100) -> ()  [unwired: 1 out]
    n153 = call <vilib>:"WPI_EncoderGet.vi"("EncoderDevRef"=w272) -> ("Distance"=→"Arm Encoder":dbl, "EncoderDevRef"=w267:T11)  [unwired: 5 in, 4 out]
    n154 = call <vilib>:"WPI_EncoderGet.vi"("EncoderDevRef"=w268) -> ("Distance"=→"stage 1 encoder":dbl, "EncoderDevRef"=w264:T11)  [unwired: 5 in, 4 out]
    n155 = call <vilib>:"WPI_EncoderGet.vi"("EncoderDevRef"=w263) -> ("Distance"=→"stage 2 encoder":dbl, "EncoderDevRef"=w262:T11)  [unwired: 5 in, 4 out]
    n156 = case shown="True" "Stage1_EncoderReset" {
      tunnel: w264 -> [_ w277]
      frame False {
      }
      frame True {
        n157 = call <vilib>:"WPI_EncoderReset.vi"("EncoderDevRef"=w277) -> ()  [unwired: 9 in, 2 out]
      }
    }
    n158 = case shown="True" "Stage2_EnconderReset" {
      tunnel: w262 -> [_ w278]
      frame False {
      }
      frame True {
        n159 = call <vilib>:"WPI_EncoderReset.vi"("EncoderDevRef"=w278) -> ()  [unwired: 9 in, 2 out]
      }
    }
    n160 = case shown="True" "Reset Enconder Arm" {
      tunnel: w267 -> [_ w279]
      frame False {
      }
      frame True {
        n161 = call <vilib>:"WPI_EncoderReset.vi"("EncoderDevRef"=w279) -> ()  [unwired: 9 in, 2 out]
      }
    }
  }
  n162 = call <vilib>:"WPI_MotorControlRefNum Registry Get.vi"("refnum name"="Shooter_ArmMotor") -> ("MotorControlDevRef"=w1:T6)  [unwired: 9 in, 1 out]
  n163 = call <vilib>:"WPI_SolenoidRefNum Registry Get.vi"("refnum name"="HatchManipulator") -> ("SolenoidDevRef"=w31:T15)  [unwired: 9 in, 1 out]
  n164 = while {
    tunnel: w31 -> [w281]
    tunnel: w1 -> [w280]
    stop <- FALSE stop-if-true
    # "When button 1 (the trigger is pressed, depending on the current position (if you are scoring\nthe ball or the hatch, the wheels spin or the pistons fire."
    n165 = global read "Robot Global Data.vi" "DriveControllerButton1_input"() -> (w282:bool)
    n166 = Wait (ms)(milliseconds to wait=u32 50) -> ()  [unwired: 1 out]
    n167 = case shown="True" w282 {
      selector: w282 -> [_ w290]
      tunnel: w281 -> [_ w287]
      tunnel: w280 -> [_ w285]
      frame False {
      }
      frame True {
        n168 = global read "Robot Global Data.vi" "Lift Position_Desired"() -> (w292:string)
        n169 = xnode "Match Regular Expression"("input string"=w292, "regular expression"="Ball") -> ("whole match"=w289:string)  [unwired: 4 in, 4 out]
        n170 = Equal?(x=w289, y="") -> (x = y?=w291:bool)
        n171 = case shown="True" w291 {
          tunnel: w290 -> [w296 w304]
          tunnel: w287 -> [_ w303]
          tunnel: w285 -> [w295 _]
          frame False {
            n172 = while {
              tunnel: w296 -> [w300]
              tunnel: w295 -> [w299]
              tunnel: [w297] -> w294
              stop <- w300 continue-if-true
              n173 = call <vilib>:"WPI_MotorControlSetOutput.vi"("Output"="Shooter Speed", "MotorControlDevRef"=w299) -> ("MotorControlDevRef"=w297:T6)  [unwired: 7 in, 2 out]
            }
            n174 = call <vilib>:"WPI_MotorControlSetOutput.vi"("Output"=0.0, "MotorControlDevRef"=w294) -> ()  [unwired: 7 in, 3 out]
          }
          frame True {
            # "You are scoring a hatch, so activate\npiston."
            n175 = while {
              tunnel: w304 -> [w307]
              tunnel: w303 -> [w308]
              tunnel: [w305] -> w301
              stop <- w307 continue-if-true
              n176 = call-poly <vilib>:"WPI_SolenoidSet.vi"("Value"=WPI_SolenoidValue."Forward", "SolenoidDevRef"=w308) -> ("SolenoidDevRef"=w305:T15)  [unwired: 8 in, 1 out]
              n177 = Wait (ms)(milliseconds to wait=u32 50) -> ()  [unwired: 1 out]
            }
            n178 = call-poly <vilib>:"WPI_SolenoidSet.vi"("Value"=WPI_SolenoidValue."Reverse", "SolenoidDevRef"=w301) -> ()  [unwired: 8 in, 2 out]
          }
        }
      }
    }
  }
  "error out" <- "error in"
